vi "set message ID.vi"(11 "request in":T1) -> (3 "request out":T1)   [LabVIEW 2013, in "Standard Engine Runtime.lvclass"]
uses:
  Standard Engine Runtime.lvclass
  main engine/message to engine.ctl
  main engine/message request type.ctl
  main engine/main engine.lvlib
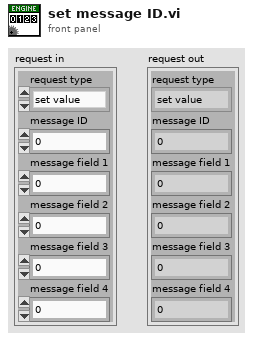
[diagram p1: front panel]
types:
  T1 = typedef "main engine.lvlib/message to engine.ctl" = cluster{"request type":T2, "message ID":u8, "message field 1":u64, "message field 2":u64, "message field 3":u64, "message field 4":u64}
  T2 = typedef "main engine.lvlib/message request type.ctl" = enum8{"set value", "disable module", "enable module"}
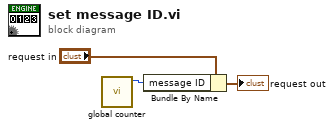
[diagram p0: block diagram]
diagram:
  n1 = call "global counter.vi"() -> ("message ID"=w3:u8)  [unwired: 11 in]
  n2 = Bundle By Name(cluster="request in", "message ID"=w3) -> (→"request out":T1)
